vi "Last Hot.vi"(10 "Threshold":u32=100, 11 "Distances":T3(array[cluster])) -> (3 "Hot Target":T2)   [LabVIEW 2013]
uses:
  Program Files (x86)/National Instruments/LabVIEW 2013/examples/FRC/Vision/2014 Target Detection/TargetType.ctl
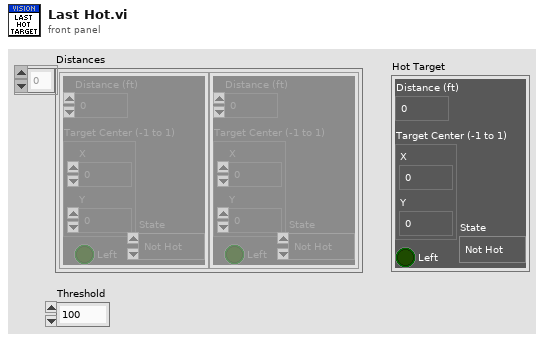
[diagram p1: front panel]
types:
  T1 = typedef "TargetType.ctl" = enum16{"Not Hot", "Hot"}
  T2 = cluster{"Distance (ft)":dbl, "Target Center (-1 to 1)":cluster{"X":dbl, "Y":dbl}, "Left":bool, "State":T1}
  T3 = cluster{"Distance (ft)":dbl, "Target Center (-1 to 1)":cluster{"X":dbl, "Y":dbl}, "Left":bool, "State":T1}[]
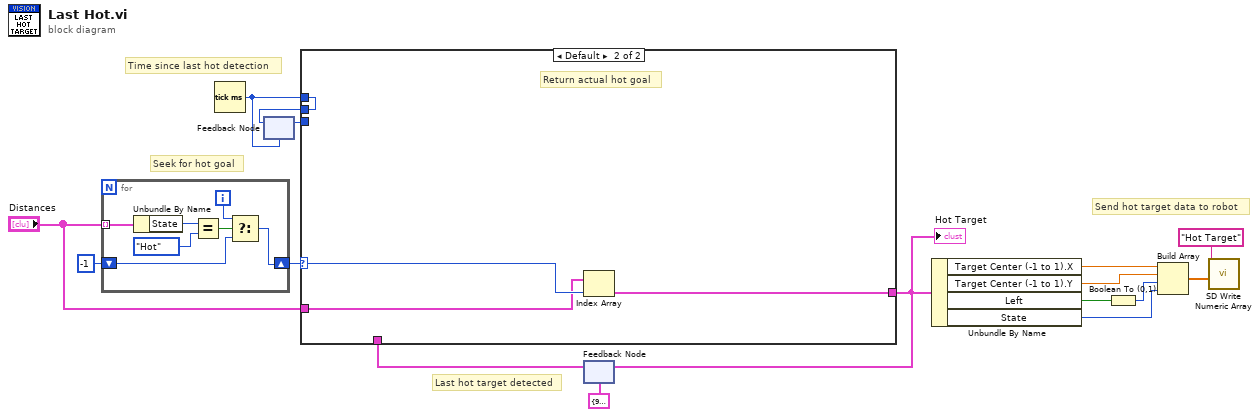
[diagram p0: block diagram]
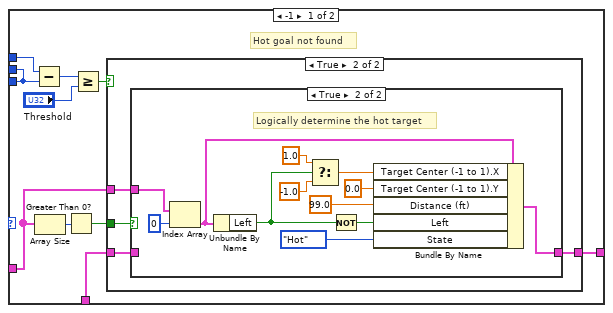
[diagram p2: hidden frame]
diagram:
  # "Last hot target detected"
  # "Time since last hot detection"
  # "Send hot target data to robot"
  # "Seek for hot goal"
  n1 = for {
    shift-right: [w18] -> w13
    shift-left: -1 -> [w19]
    tunnel: "Distances" -> [w17] mode=indexing
    i -> [w21]
    n2 = Unbundle By Name(w17) -> ("State"=w22:T1)
    n3 = Equal?(x=w22, y=TargetType."Hot") -> (x = y?=w20:bool)
    n4 = Select(t=w21, s=w20, f=w19) -> (s? t:f=w18:i32)
  }
  n5 = Tick Count (ms)() -> (millisecond timer value=w14:u32)
  n6 = feedback #1(w14) -> (w15:u32)
  n7 = feedback #2(T2 {"Distance (ft)"=99.0, "Target Center (-1 to 1)"={"X"=1.0, "Y"=1.0}, "Left"=FALSE, "State"=enum."Not Hot"}) -> (w9:T2)
  n8 = case shown="Default" w13 {
    selector: w13 -> [_ w55]
    tunnel: w15 -> [w24 _]
    tunnel: w14 -> [w31 w52]
    tunnel: "Distances" -> [w25 w54]
    tunnel: [w27 w53] -> w8
    tunnel: w9 -> [w28 _]
    tunnel: [w24 w52] -> w1
    frame -1 {
      # "Hot goal not found"
      n9 = Subtract(x=w31, y=w24) -> (x-y=w33:u32)
      n10 = Array Size(array=w25) -> (size(s)=w29:i32)
      n11 = Greater Than 0?(x=w29) -> (x > 0?=w26:bool)
      n12 = Greater Or Equal?(x=w33, y="Threshold") -> (x >= y?=w30:bool)
      n13 = case shown="True" w30 {
        tunnel: w28 -> [w34 w36]
        tunnel: [w34 w35] -> w27
        tunnel: w26 -> [_ w38]
        tunnel: w25 -> [_ w37]
        frame False {
          # "Time fits in threshold, return last hot target"
        }
        frame True {
          n14 = case shown="True" w38 {
            tunnel: w37 -> [_ w51]
            tunnel: w36 -> [w39 _]
            tunnel: [w39 w40] -> w35
            frame False {
              # "Out of options, return last hot target"
            }
            frame True {
              # "Logically determine the hot target"
              n15 = Index Array(array=w51, index=0) -> (element=w49:T2)
              n16 = Unbundle By Name(w49) -> ("Left"=w43:bool)
              n17 = Select(t=1.0, s=w43, f=-1.0) -> (s? t:f=w44:dbl)
              n18 = Not(x=w43) -> (.not. x?=w50:bool)
              n19 = Bundle By Name(cluster=w49, "Target Center (-1 to 1).X"=w44, "Target Center (-1 to 1).Y"=0.0, "Distance (ft)"=99.0, "Left"=w50, "State"=TargetType."Hot") -> (w40:T2)
            }
          }
        }
      }
    }
    frame Default {
      # "Return actual hot goal"
      n20 = Index Array(array=w54, index=w55) -> (element=w53:T2)
    }
  }
  "Hot Target" <- w8
  n21 = feedback-in #1(w1) -> ()
  n22 = feedback-in #2(w8) -> ()
  n23 = Unbundle By Name(w8) -> ("Target Center (-1 to 1).X"=w6:dbl, "Target Center (-1 to 1).Y"=w5:dbl, "Left"=w7:bool, "State"=w4:T1)
  n24 = Boolean To (0,1)(Boolean=w7) -> (0, 1=w11:i16)
  n25 = Build Array(w6, w5, w11, w4) -> (w3:dbl[])
  n26 = call <vilib>:"SD Write Numeric Array.vi"("Numeric Array"=w3, "Name"="Hot Target") -> ()  [unwired: 8 in, 2 out]
